vi "parse bmp.vi"(8 "error in (no error)":errorcluster, 11 "<bmp> string":string) -> (0 "error out":errorcluster, 3 "bmp data":T1)   [LabVIEW 2018, in "Data Parser.lvclass"]
uses:
  Data Parser.lvclass
  Bmp data.ctl
  Bmp File Data.ctl
panel:
  out "debug array":string[](array[string])
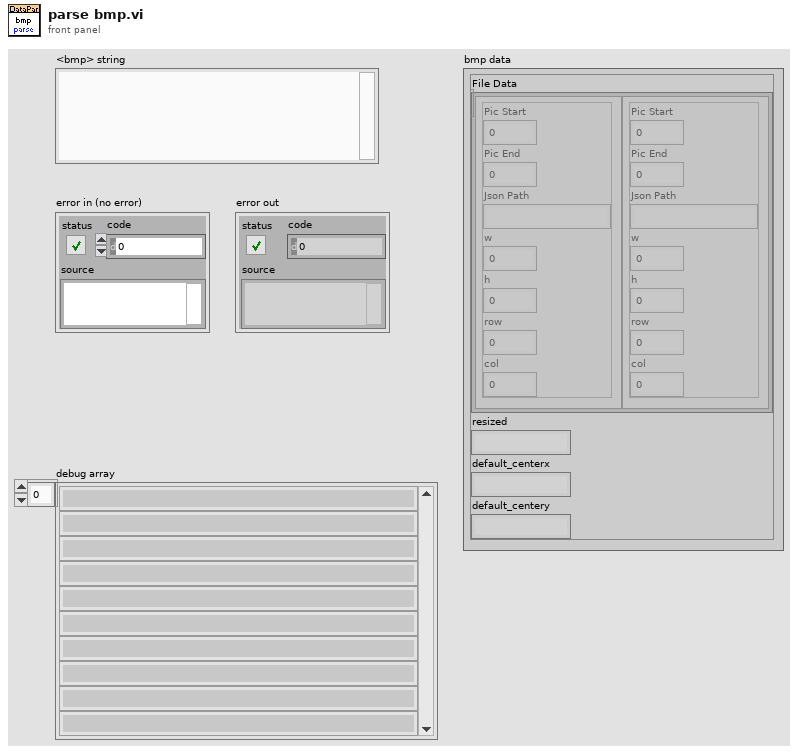
[diagram p1: front panel]
types:
  T1 = typedef "Data Parser.lvclass/Bmp data.ctl" = cluster{"File Data":T2[], "resized":string, "default_centerx":string, "default_centery":string}
  T2 = typedef "Data Parser.lvclass/Bmp File Data.ctl" = cluster{"Pic Start":i32, "Pic End":i32, "Json Path":string, "w":i32, "h":i32, "row":i32, "col":i32}
  T3 = cluster{"pic start":i32, "pic end":i32, "json path":string, "w":i32, "h":i32, "row":i32, "col":i32}
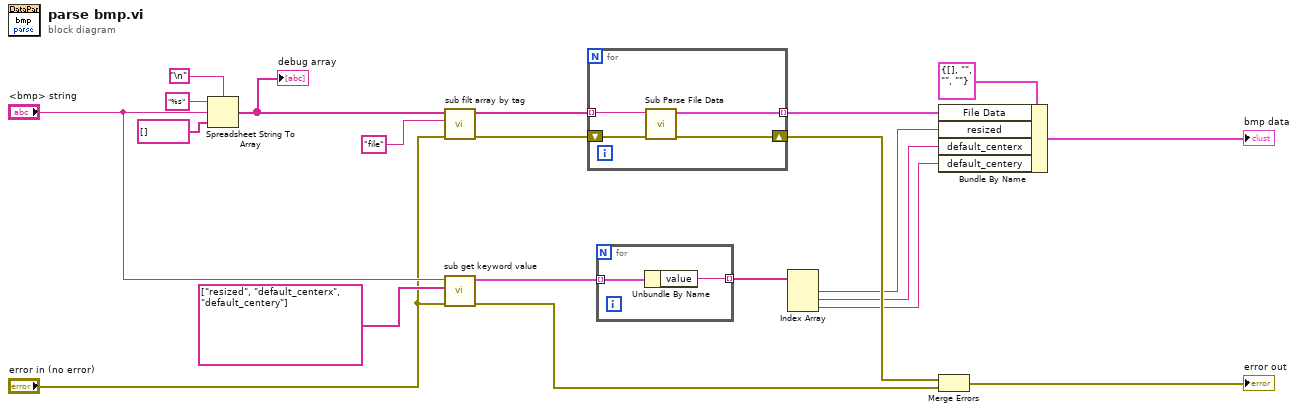
[diagram p0: block diagram]
diagram:
  n1 = Spreadsheet String To Array(delimiter (Tab)="\n", format string="%s", spreadsheet string="<bmp> string", array type (2D Dbl)=string[] []) -> (array=w18:string[])
  "debug array" <- w18
  n2 = call "sub filt array by tag.vi"("error in"="error in (no error)", "tag"="file" ("String"), "string array"=w18) -> ("error out"=w12:errorcluster, "filted string array"=w16:string[])  [unwired: 7 in]
  n3 = call "sub get keyword value.vi"("error in"="error in (no error)", "keyword"=string[] ["resized", "default_centerx", "default_centery"], "string"="<bmp> string") -> ("error out"=w7:errorcluster, "matched pairs (all)"=w5:cluster{"keyword":string, "value":string}[])  [unwired: 5 in, 2 out]
  n4 = for {
    tunnel: [w25] -> w14 mode=indexing
    tunnel: w16 -> [w24] mode=indexing
    shift-right: [w22] -> w8
    shift-left: w12 -> [w23]
    n5 = call "Sub Parse File Data.vi"("error in (no error)"=w23, "input string"=w24) -> ("error out"=w22:errorcluster, "file data"=w25:T3)  [unwired: 8 in]
  }
  n6 = for {
    tunnel: w5 -> [w27] mode=indexing
    tunnel: [w26] -> w4 mode=indexing
    n7 = Unbundle By Name(w27) -> ("value"=w26:string)
  }
  n8 = Index Array(array=w4) -> (element #1=w3:string, element #2=w2:string, element #3=w1:string)  [unwired: 3 in]
  n9 = Bundle By Name(cluster=T1 {"File Data"=[], "resized"="", "default_centerx"="", "default_centery"=""} ("bmp data"), "File Data"=w14, "resized"=w3, "default_centerx"=w2, "default_centery"=w1) -> (→"bmp data":T1)
  n10 = Merge Errors(w8, w7) -> (→"error out":errorcluster)
